vi "Load_SampleImage.vi"(8 "error in":errorcluster caption="entrée d'erreur", 11 "Image":u16(ring) items=["China", "Flower"]) -> (0 "error out":errorcluster caption="sortie d'erreur", 3 "Image (RGB)":string[][](array[string]))   [LabVIEW 2020]
doc: "Scikit-learn also embed a couple of sample JPEG images published under Creative Commons license by their authors. Those images can be useful to test algorithms and pipeline on 2D data.\n\nLoad sample images for image manipulation. Loads both, china and flower.\n\nimages : list of ndarray of shape (427, 640, 3) (height x width x color(RGB))"
uses:
  Load_SampleImage.lvclass
panel:
  out "Load_SampleImage en entrée":refnum<class "Load_SampleImage.lvclass">
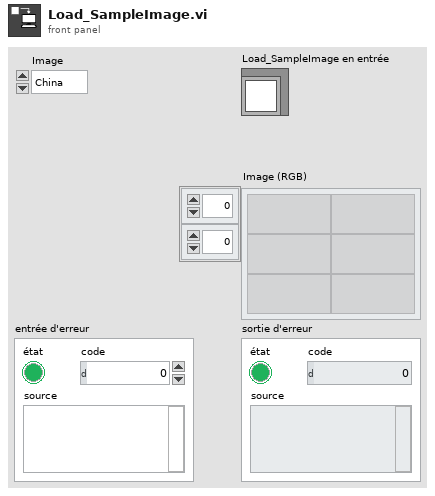
[diagram p1: front panel]
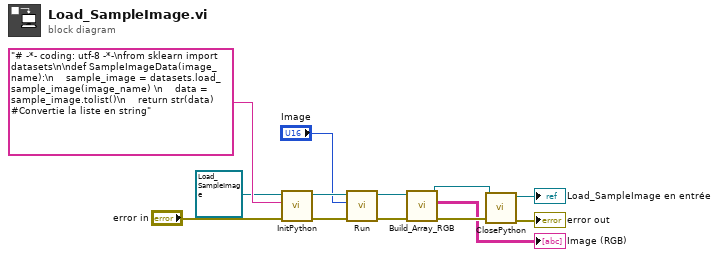
[diagram p0: block diagram]
diagram:
  n1 = call-dynamic "InitPython.vi"("error in (no error)"="error in", "Python Instruction"="# -*- coding: utf-8 -*-\nfrom sklearn import datasets\n\ndef SampleImageData(image_name):\n    sample_image = datasets.load_sample_image(image_name) \n    data = sample_image.tolist()\n    return str(data) #Convertie la liste en string", "Scikit-learn en entrée"=refnum<class "Load_SampleImage.lvclass"> refnum ("Load_SampleImage.lvclass")) -> ("error out"=w10:errorcluster, "Scikit-learn en sortie"=w8:refnum<class "Load_SampleImage.lvclass">)  [unwired: 7 in]
  n2 = call-dynamic "Run.vi"("error in (no error)"=w10, "Image"="Image", "Load_SampleImage en entrée"=w8) -> ("error out"=w6:errorcluster, "Load_SampleImage en entrée"=w7:refnum<class "Load_SampleImage.lvclass">)  [unwired: 7 in]
  n3 = call-dynamic "Build_Array_RGB.vi"("error in (no error)"=w6, "Load_SampleImage en entrée"=w7) -> ("error out"=w4:errorcluster, "Image (RGB)"=→"Image (RGB)":string[][], "Load_SampleImage en entrée"=w5:refnum<class "Load_SampleImage.lvclass">)  [unwired: 7 in]
  n4 = call-dynamic "ClosePython.vi"("error in (no error)"=w4, "Scikit-learn en entrée"=w5) -> ("error out"=→"error out":errorcluster, "Scikit-learn en sortie"=→"Load_SampleImage en entrée":refnum<class "Load_SampleImage.lvclass">)  [unwired: 8 in]
